vi "Struct Fill Cluster By Items Record.vi"(7 "reinit cluster to default (false)":bool, 8 "error in":errorcluster, 9 "data start offset (0)":i32, 10 "data in":u8[](array[numeric])=[9, 0, 0, 0, 15, 0, 0, 0, 1, 78, 0, 1, 0, 0, 0, 1, 0, 0, 0, 1, 0, 0, 0, 43, 0, 0, 0, 1, 97, 3, 1, 0, 0, 0, 4, 0, 0, 0, 0, 0, 0, 0, 0, 0, 240, 63, 0, 0, 0, 0, 0, 0, 0, 64, 0, 0, 0, 0, 0, 0, 8, 64, 0, 0, 0, 0, 0, 0, 16, 64, 43, 0, 0, 0, 1, 66, 3, 2, 0, 0, 0, 2, 0, 0, 0, 0, 0, 0, 0, 0, 0, 240, 63, 0, 0, 0, 0, 0, 0, 8, 64, 0, 0, 0, 0, 0, 0, 0, 64, 0, 0, 0, 0, 0, 0, 16, 64, 22, 0, 0, 0, 3, 115, 116, 114, 4, 1, 0, 0, 0, 9, 0, 0, 0, 100, 118, 101, 32, 104, 111, 118, 110, 111, 44, 0, 0, 0, 2, 99, 97, 131, 2, 0, 0, 0, 1, 0, 0, 0, 0, 0, 0, 0, 0, 0, 240, 63, 0, 0, 0, 0, 0, 0, 240, 63, 0, 0, 0, 0, 0, 0, 0, 64, 0, 0, 0, 0, 0, 0, 240, 191, 109, 0, 0, 0, 5, 115, 116, 114, 117, 99, 5, 1, 0, 0, 0, 1, 0, 0, 0, 3, 0, 0, 0, 16, 0, 0, 0, 3, 115, 116, 114, 4, 1, 0, 0, 0, 3, 0, 0, 0, 97, 115, 115, 19, 0, 0, 0, 1, 110, 3, 1, 0, 0, 0, 1, 0, 0, 0, 0, 0, 0, 0, 0, 128, 75, 64, 43, 0, 0, 0, 1, 65, 3, 2, 0, 0, 0, 2, 0, 0, 0, 0, 0, 0, 0, 0, 0, 240, 63, 0, 0, 0, 0, 0, 0, 8, 64, 0, 0, 0, 0, 0, 0, 0, 64, 0, 0, 0, 0, 0, 0, 16, 64, 218, 0, 0, 0, 2, 115, 118, 5, 1, 0, 0, 0, 2, 0, 0, 0, 3, 0, 0, 0, 16, 0, 0, 0, 3, 115, 116, 114, 4, 1, 0, 0, 0, 3, 0, 0, 0, 97, 115, 115, 19, 0, 0, 0, 1, 110, 3, 1, 0, 0, 0, 1, 0, 0, 0, 0, 0, 0, 0, 0, 128, 75, 64, 43, 0, 0, 0, 1, 65, 3, 2, 0, 0, 0, 2, 0, 0, 0, 0, 0, 0, 0, 0, 0, 240, 63, 0, 0, 0, 0, 0, 0, 8, 64, 0, 0, 0, 0, 0, 0, 0, 64, 0, 0, 0, 0, 0, 0, 16, 64, 3, 0, 0, 0, 34, 0, 0, 0, 3, 115, 116, 114, 4, 1, 0, 0, 0, 21, 0, 0, 0, 110, 101, 106, 97, 107, 101, 106, 32, 106, 105, 110, 101, 106, 32, 114, 101, 116, 101, 122, 101, 99, 19, 0, 0, 0, 1, 110, 3, 1, 0, 0, 0, 1, 0, 0, 0, 0, 0, 0, 0, 0, 0, 86, 64, 43, 0, 0, 0, 1, 65, 3, 2, 0, 0, 0, 2, 0, 0, 0, 0, 0, 0, 0, 0, 0, 240, 63, 0, 0, 0, 0, 0, 0, 8, 64, 0, 0, 0, 0, 0, 0, 0, 64, 0, 0, 0, 0, 0, 0, 16, 64, 132, 1, 0, 0, 2, 115, 99, 5, 2, 0, 0, 0, 2, 0, 0, 0, 3, 0, 0, 0, 16, 0, 0, 0, 3, 115, 116, 114, 4, 1, 0, 0, 0, 3, 0, 0, 0, 97, 115, 115, 19, 0, 0, 0, 1, 110, 3, 1, 0, 0, 0, 1, 0, 0, 0, 0, 0, 0, 0, 0, 128, 75, 64, 43, 0, 0, 0, 1, 65, 3, 2, 0, 0, 0, 2, 0, 0, 0, 0, 0, 0, 0, 0, 0, 240, 63, 0, 0, 0, 0, 0, 0, 8, 64, 0, 0, 0, 0, 0, 0, 0, 64, 0, 0, 0, 0, 0, 0, 16, 64, 3, 0, 0, 0, 16, 0, 0, 0, 3, 115, 116, 114, 4, 1, 0, 0, 0, 3, 0, 0, 0, 97, 115, 115, 19, 0, 0, 0, 1, 110, 3, 1, 0, 0, 0, 1, 0, 0, 0, 0, 0, 0, 0, 0, 128, 75, 64, 43, 0, 0, 0, 1, 65, 3, 2, 0, 0, 0, 2, 0, 0, 0, 0, 0, 0, 0, 0, 0, 240, 63, 0, 0, 0, 0, 0, 0, 8, 64, 0, 0, 0, 0, 0, 0, 0, 64, 0, 0, 0, 0, 0, 0, 16, 64, 3, 0, 0, 0, 16, 0, 0, 0, 3, 115, 116, 114, 4, 1, 0, 0, 0, 3, 0, 0, 0, 97, 115, 115, 19, 0, 0, 0, 1, 110, 3, 1, 0, 0, 0, 1, 0, 0, 0, 0, 0, 0, 0, 0, 128, 75, 64, 43, 0, 0, 0, 1, 65, 3, 2, 0, 0, 0, 2, 0, 0, 0, 0, 0, 0, 0, 0, 0, 240, 63, 0, 0, 0, 0, 0, 0, 8, 64, 0, 0, 0, 0, 0, 0, 0, 64, 0, 0, 0, 0, 0, 0, 16, 64, 3, 0, 0, 0, 16, 0, 0, 0, 3, 115, 116, 114, 4, 1, 0, 0, 0, 3, 0, 0, 0, 97, 115, 115, 19, 0, 0, 0, 1, 110, 3, 1, 0, 0, 0, 1, 0, 0, 0, 0, 0, 0, 0, 0, 128, 75, 64, 43, 0, 0, 0, 1, 65, 3, 2, 0, 0, 0, 2, 0, 0, 0, 0, 0, 0, 0, 0, 0, 240, 63, 0, 0, 0, 0, 0, 0, 8, 64, 0, 0, 0, 0, 0, 0, 0, 64, 0, 0, 0, 0, 0, 0, 16, 64, 26, 0, 0, 0, 4, 99, 115, 116, 114, 5, 1, 0, 0, 0, 3, 0, 0, 0, 0, 0, 0, 0, 0, 0, 0, 0, 0, 0, 0, 0], 11 "cluster ref (empty)":refnum<vi>) -> (0 "error out":errorcluster, 2 "octave struct out":T1[](array[typedef]), 3 "cluster ref out (copy)":refnum<vi>)   [LabVIEW 2013, in "GOLPI library.lvlib"]
doc: "This VI will use binary struct data generated by GNU Octave GOLPI function 'golpi_conv_struct()'. It will try to assign all elements from the Octave to the elements of matching names in the referenced cluser. Optionally it can reset the cluster default before. If it is called with invalid reference to the cluster it will just parse the binary data and return the items list. The function is recoursive so it should be able to assign clusters within clusters and so on."
uses:
  GOLPI library.lvlib
  Struct Item Record.ctl
  Struct Item Types.ctl
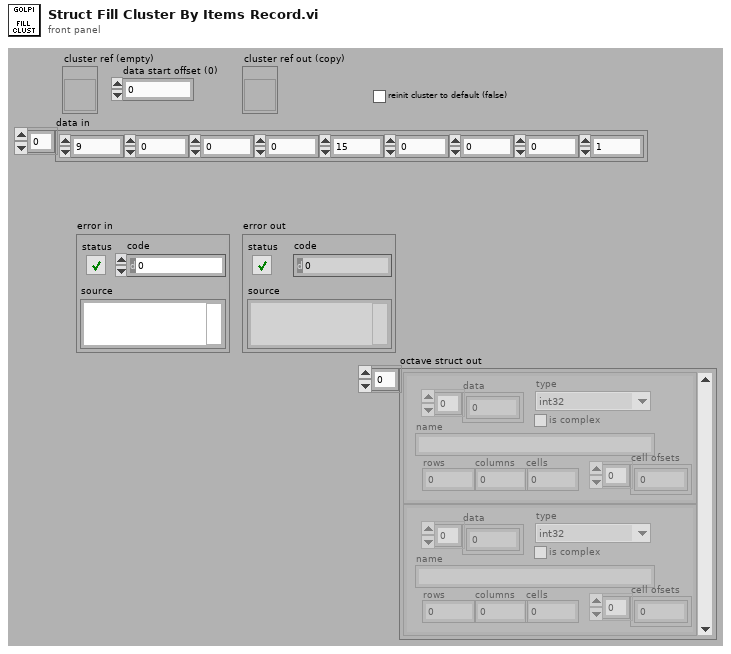
[diagram p1: front panel]
types:
  T1 = typedef "GOLPI library.lvlib/Struct Item Record.ctl" = cluster{"data":u8[], "type":T2, "name":string, "rows":i32, "columns":i32, "cells":i32, "is complex":bool, "cell ofsets":u32[]}
  T2 = typedef "GOLPI library.lvlib/Struct Item Types.ctl" = enum16{"int32", "uint32", "single", "double", "string", "cell array"}
  T3 = enum16{"big-endian, network order", "native, host order", "little-endian"}
  T4 = typedef "GOLPI library.lvlib/Struct Data Types.ctl" = enum16{"n/a", "Real", "Complex", "String/path", "Cluster", "Bool"}
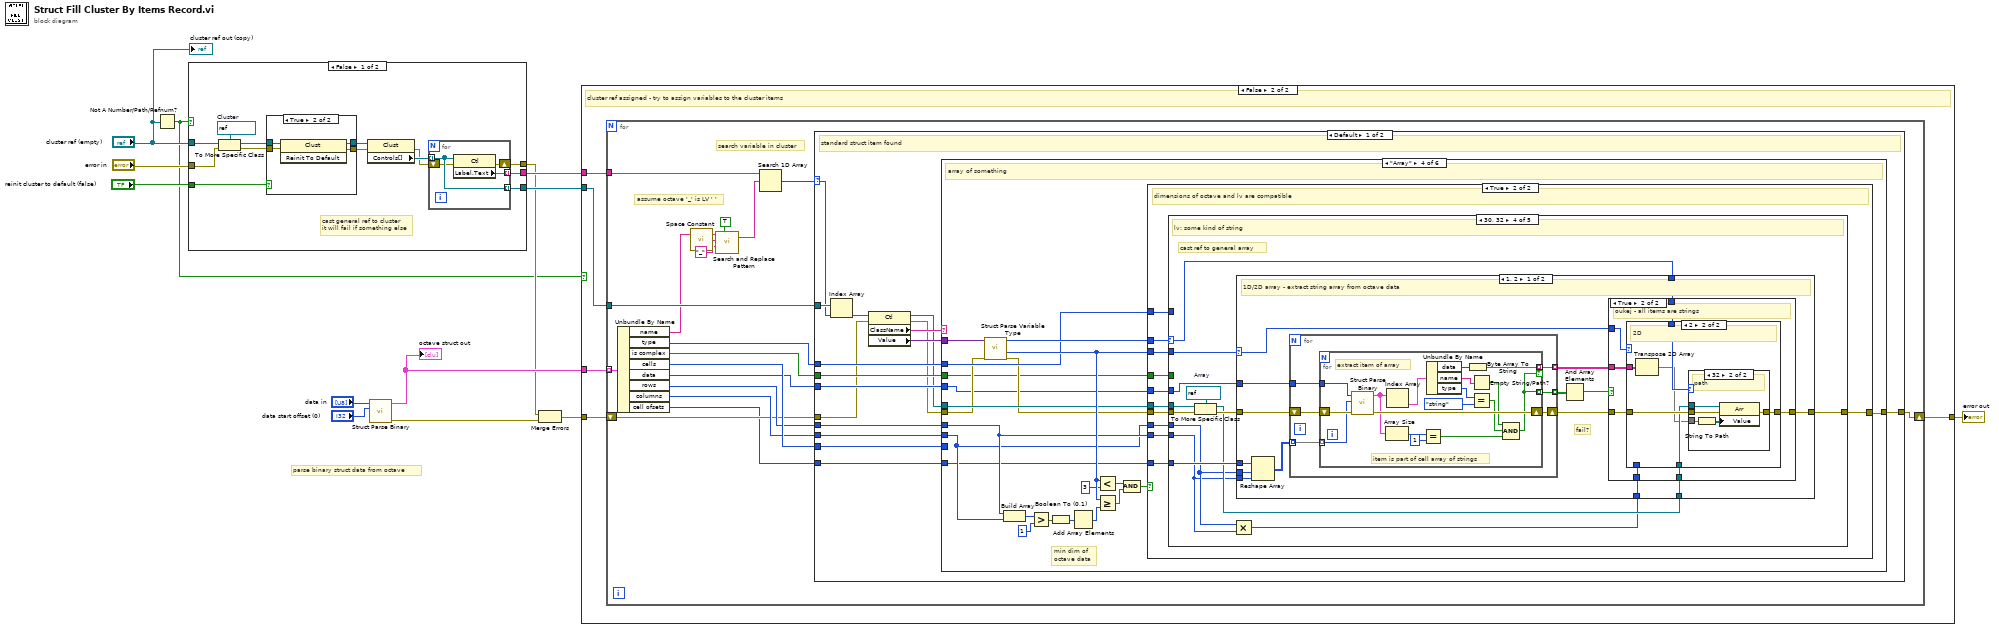
[diagram p0: block diagram]
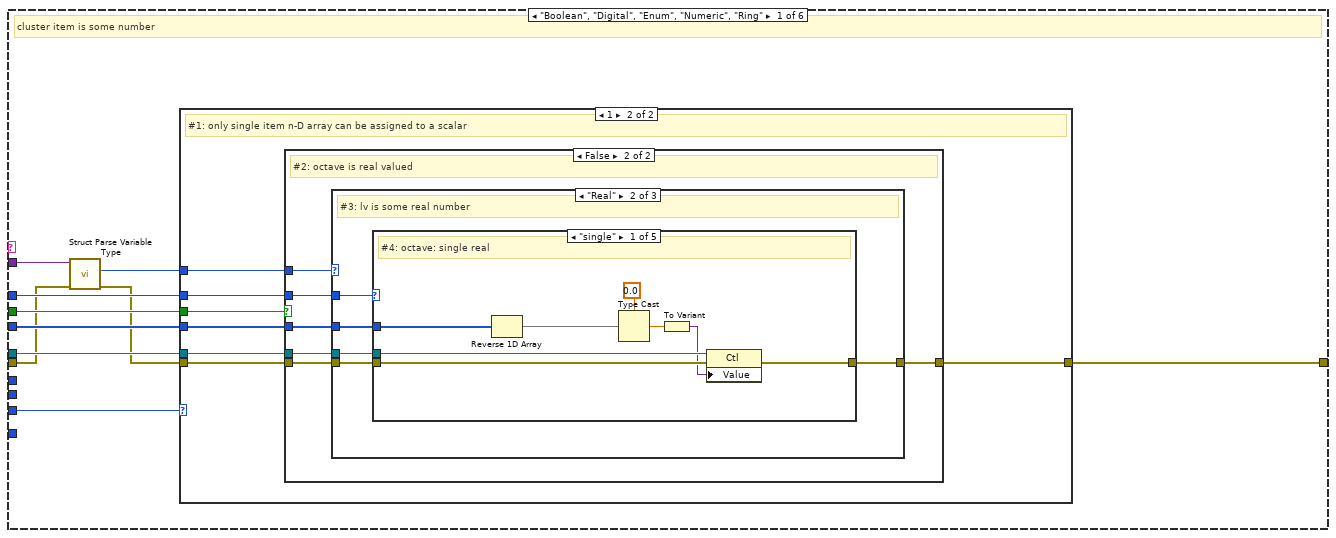
[diagram p3: hidden frame]
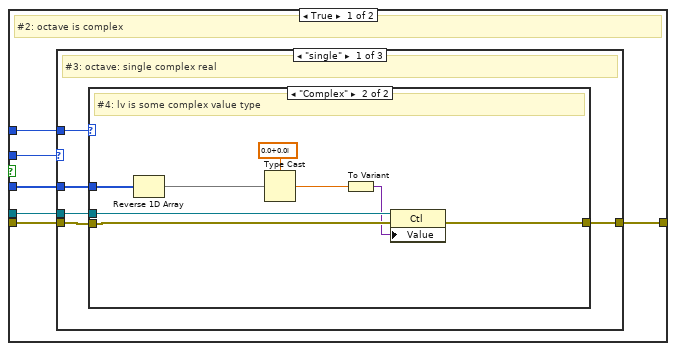
[diagram p5: hidden frame]
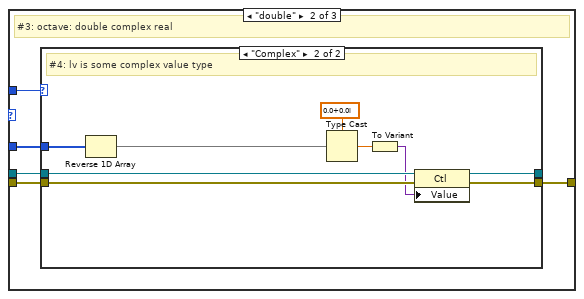
[diagram p7: hidden frame]
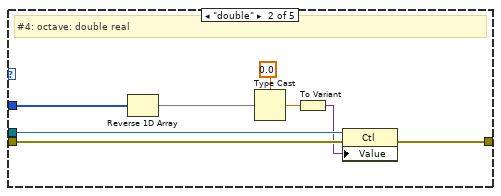
[diagram p11: hidden frame]
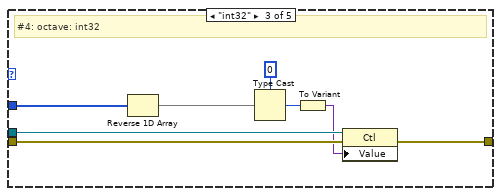
[diagram p12: hidden frame]
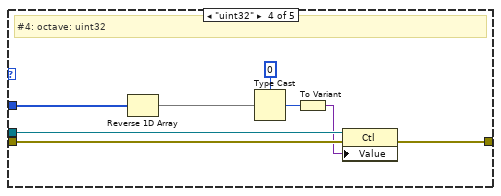
[diagram p13: hidden frame]
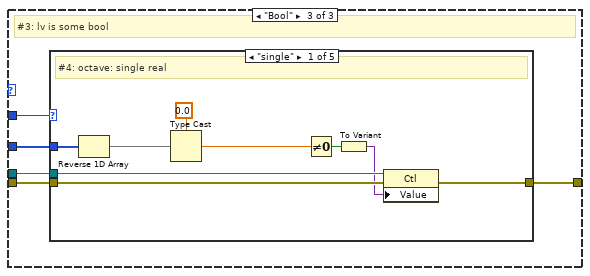
[diagram p15: hidden frame]
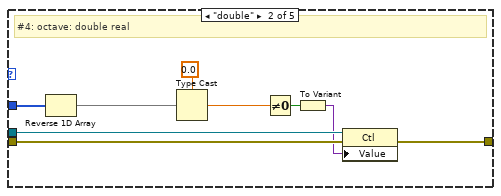
[diagram p16: hidden frame]
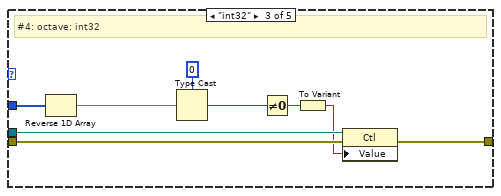
[diagram p17: hidden frame]
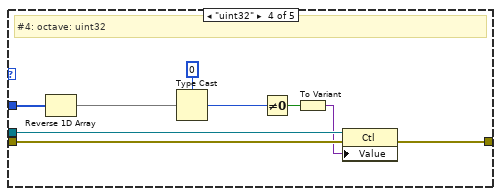
[diagram p18: hidden frame]
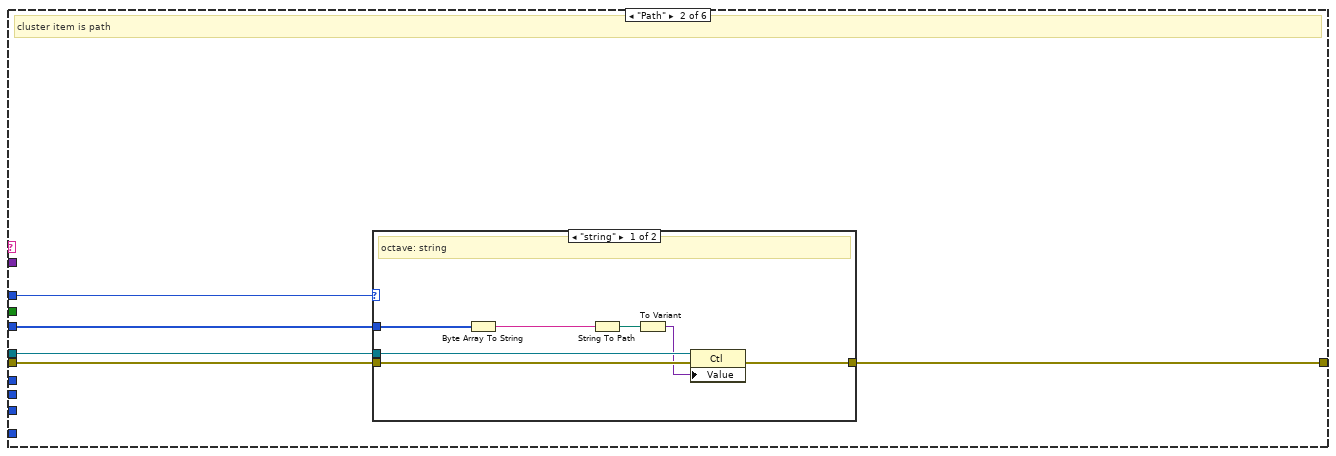
[diagram p20: hidden frame]
diagram:
  # "parse binary struct data from octave"
  n1 = Not A Number/Path/Refnum?(number/path/refnum="cluster ref (empty)") -> (NaN/Path/Refnum?=w1:bool)
  n2 = case shown="False" w1 {
    tunnel: [w25 _] -> w11
    tunnel: [w24 _] -> w10
    tunnel: "error in" -> [w22 w37]
    tunnel: "cluster ref (empty)" -> [w15 _]
    tunnel: "reinit cluster to default (false)" -> [w17 _]
    tunnel: [w14 w37] -> w4
    frame False {
      w23 = refnum<vi> refnum  # Cluster
      # "cast general ref to cluster\nit will fail if something else"
      n3 = To More Specific Class(target class=w23, reference=w15, error in=w22) -> (specific class reference=w19:refnum<vi>, error out=w18:errorcluster)
      n4 = case shown="True" w17 {
        tunnel: [w28 w32] -> w21
        tunnel: [w27 w31] -> w20
        tunnel: w19 -> [w27 w30]
        tunnel: w18 -> [w28 w29]
        frame False {
        }
        frame True {
          n5 = invoke class="Clust" method="Reinit To Default"(reference=w30, error in=w29) -> (reference out=w31:refnum<vi>, error out=w32:errorcluster)  [unwired: 1 in, 1 out]
        }
      }
      n6 = property class="Clust"(reference=w20, error in=w21) -> (error out=w16:errorcluster, "Controls[]"=w26:refnum<vi>[])  [unwired: 1 out]
      n7 = for {
        tunnel: w26 -> [w35] mode=indexing
        tunnel: [w36] -> w25 mode=indexing
        tunnel: [w35] -> w24 mode=indexing
        shift-right: [w33] -> w14
        shift-left: w16 -> [w34]
        n8 = property class="Ctl"(reference=w35, error in=w34) -> (error out=w33:errorcluster, "Label.Text"=w36:string)  [unwired: 1 out]
      }
    }
    frame True {
    }
  }
  n9 = call "Struct Parse Binary.vi"("data start offset (0)"="data start offset (0)", "data in"="data in") -> ("error out"=w3:errorcluster, "struct items"=w12:T1[])  [unwired: 8 in]
  "octave struct out" <- w12
  n10 = Merge Errors(w4, w3) -> (w2:errorcluster)
  n11 = case shown="False" w1 {
    tunnel: w12 -> [_ w43]
    tunnel: w11 -> [_ w42]
    tunnel: w10 -> [_ w41]
    tunnel: [w38 w40] -> w9
    tunnel: w2 -> [w38 w39]
    frame True {
      # "no cluster ref assigned - skip assigning, just parse struct"
    }
    frame False {
      # "cluster ref assigned - try to assign variables to the cluster items"
      n12 = for {
        tunnel: w43 -> [w61] mode=indexing
        tunnel: w42 -> [w60]
        tunnel: w41 -> [w59]
        shift-right: [w52] -> w40
        shift-left: w39 -> [w51]
        # "assume octave '_' is LV ' '"
        # "search variable in cluster"
        n13 = Unbundle By Name(w61) -> ("name"=w48:string, "type"=w58:T2, "is complex"=w57:bool, "cells"=w56:i32, "data"=w55:u8[], "rows"=w54:i32, "columns"=w53:i32, "cell ofsets"=w50:u32[])
        n14 = call <vilib>:"Space Constant.vi"() -> ("String"=w44:string)
        n15 = call <vilib>:"Search and Replace Pattern.vi"("string"=w48, "regular expression (\"\")"="_", "replace string (\"\")"=w44, "replace all? (F)"=TRUE) -> ("result string"=w47:string)  [unwired: 1 in, 1 out]
        n16 = Search 1D Array(1D array=w60, element=w47) -> (index of element=w49:i32)  [unwired: 1 in]
        n17 = case shown="Default" w49 {
          selector: w49 -> [w76 _]
          tunnel: w59 -> [w77 _]
          tunnel: w58 -> [w72 _]
          tunnel: w57 -> [w71 _]
          tunnel: w56 -> [w70 _]
          tunnel: w55 -> [w69 _]
          tunnel: w54 -> [w66 _]
          tunnel: w53 -> [w65 _]
          tunnel: [w64 w626] -> w52
          tunnel: w51 -> [w63 w626]
          tunnel: w50 -> [w62 _]
          frame Default {
            # "standard struct item found"
            n18 = Index Array(array=w77, index=w76) -> (element=w75:refnum<vi>)
            n19 = property class="Ctl"(reference=w75, error in=w63) -> (reference out=w68:refnum<vi>, error out=w67:errorcluster, "ClassName"=w74:string, "Value"=w73:variant)
            n20 = case shown="\"Array\"" w74 {
              tunnel: w73 -> [w87 _ _ w246 _ _]
              tunnel: w72 -> [w86 w224 w237 w253 w613 _]
              tunnel: w71 -> [w82 _ _ w250 _ _]
              tunnel: w70 -> [w83 _ _ _ w615 _]
              tunnel: w69 -> [w85 w223 w236 w249 w607 _]
              tunnel: w68 -> [w81 w222 w235 w255 w608 _]
              tunnel: w67 -> [w79 w221 w234 w252 w616 w625]
              tunnel: [w80 w220 w233 w256 w606 w625] -> w64
              tunnel: w66 -> [_ _ _ w248 _ _]
              tunnel: w65 -> [_ _ _ w247 _ _]
              tunnel: w62 -> [_ _ _ w245 _ _]
              frame "Boolean", "Digital", "Enum", "Numeric", "Ring" {
                # "cluster item is some number"
                n21 = call "Struct Parse Variable Type.vi"("error in"=w79, "variant in"=w87) -> ("error out"=w78:errorcluster, "data type"=w84:T4)  [unwired: 6 in, 2 out]
                n22 = case shown="1" w83 {
                  tunnel: w86 -> [_ w95]
                  tunnel: w85 -> [_ w94]
                  tunnel: w84 -> [_ w93]
                  tunnel: w82 -> [_ w92]
                  tunnel: w81 -> [_ w91]
                  tunnel: w78 -> [w88 w90]
                  tunnel: [w88 w89] -> w80
                  frame Default {
                    # "error - can't assign multi cell array to a scalar"
                  }
                  frame 1 {
                    # "#1: only single item n-D array can be assigned to a scalar"
                    n23 = case shown="False" w92 {
                      tunnel: w95 -> [w101 w138]
                      tunnel: w94 -> [w100 w137]
                      tunnel: w93 -> [w99 w133]
                      tunnel: w91 -> [w98 w136]
                      tunnel: w90 -> [w97 w135]
                      tunnel: [w96 w134] -> w89
                      frame True {
                        # "#2: octave is complex"
                        n24 = case shown="\"single\"" w101 {
                          tunnel: w100 -> [w105 w119 _]
                          tunnel: w99 -> [w106 w120 _]
                          tunnel: w98 -> [w104 w118 _]
                          tunnel: w97 -> [w103 w117 w132]
                          tunnel: [w102 w116 w132] -> w96
                          frame "single" {
                            # "#3: octave: single complex real"
                            n25 = case shown="\"Complex\"" w106 {
                              tunnel: w105 -> [_ w115]
                              tunnel: w104 -> [_ w112]
                              tunnel: w103 -> [w107 w111]
                              tunnel: [w107 w108] -> w102
                              frame Default {
                                # "#4: error: invalid octave type"
                              }
                              frame "Complex" {
                                # "#4: lv is some complex value type"
                                n26 = Reverse 1D Array(array=w115) -> (reversed array=w114:u8[])
                                n27 = Type Cast(type=csg 0.0+0.0i, x=w114) -> (*(type *) &x=w110:csg)
                                n28 = To Variant(anything=w110) -> (Variant=w109:variant)
                                n29 = property class="Ctl"(reference=w112, error in=w111, "Value"=w109) -> (error out=w108:errorcluster)  [unwired: 1 out]
                              }
                            }
                          }
                          frame "double" {
                            # "#3: octave: double complex real"
                            n30 = case shown="\"Complex\"" w120 {
                              tunnel: w119 -> [_ w131]
                              tunnel: w118 -> [w121 w128]
                              tunnel: w117 -> [w122 w127]
                              tunnel: [w122 w124] -> w116
                              tunnel: [w121 w123] -> _
                              frame Default {
                              }
                              frame "Complex" {
                                # "#4: lv is some complex value type"
                                n31 = Reverse 1D Array(array=w131) -> (reversed array=w130:u8[])
                                n32 = Type Cast(type=cdb 0.0+0.0i, x=w130) -> (*(type *) &x=w126:cdb)
                                n33 = To Variant(anything=w126) -> (Variant=w125:variant)
                                n34 = property class="Ctl"(reference=w128, error in=w127, "Value"=w125) -> (reference out=w123:refnum<vi>, error out=w124:errorcluster)
                              }
                            }
                          }
                          frame Default {
                            # "#3: invalid octave type"
                          }
                        }
                      }
                      frame False {
                        # "#2: octave is real valued"
                        n35 = case shown="\"Real\"" w133 {
                          tunnel: w138 -> [_ w144 w182]
                          tunnel: w137 -> [_ w143 w181]
                          tunnel: w136 -> [_ w142 w180]
                          tunnel: w135 -> [w139 w141 w179]
                          tunnel: [w139 w140 w178] -> w134
                          frame Default {
                            # "#3: bad lv type"
                          }
                          frame "Real" {
                            # "#3: lv is some real number"
                            n36 = case shown="\"single\"" w144 {
                              tunnel: w143 -> [w152 w160 w168 w176 _]
                              tunnel: w142 -> [w151 w159 w167 w175 _]
                              tunnel: w141 -> [w150 w158 w166 w174 w177]
                              tunnel: [w149 w157 w165 w173 w177] -> w140
                              frame "single" {
                                # "#4: octave: single real"
                                n37 = Reverse 1D Array(array=w152) -> (reversed array=w148:u8[])
                                n38 = Type Cast(type=sgl 0.0, x=w148) -> (*(type *) &x=w146:sgl)
                                n39 = To Variant(anything=w146) -> (Variant=w145:variant)
                                n40 = property class="Ctl"(reference=w151, error in=w150, "Value"=w145) -> (error out=w149:errorcluster)  [unwired: 1 out]
                              }
                              frame "double" {
                                # "#4: octave: double real"
                                n41 = Reverse 1D Array(array=w160) -> (reversed array=w156:u8[])
                                n42 = Type Cast(type=0.0, x=w156) -> (*(type *) &x=w154:dbl)
                                n43 = To Variant(anything=w154) -> (Variant=w153:variant)
                                n44 = property class="Ctl"(reference=w159, error in=w158, "Value"=w153) -> (error out=w157:errorcluster)  [unwired: 1 out]
                              }
                              frame "int32" {
                                # "#4: octave: int32"
                                n45 = Reverse 1D Array(array=w168) -> (reversed array=w164:u8[])
                                n46 = Type Cast(type=0, x=w164) -> (*(type *) &x=w162:i32)
                                n47 = To Variant(anything=w162) -> (Variant=w161:variant)
                                n48 = property class="Ctl"(reference=w167, error in=w166, "Value"=w161) -> (error out=w165:errorcluster)  [unwired: 1 out]
                              }
                              frame "uint32" {
                                # "#4: octave: uint32"
                                n49 = Reverse 1D Array(array=w176) -> (reversed array=w172:u8[])
                                n50 = Type Cast(type=u32 0, x=w172) -> (*(type *) &x=w170:u32)
                                n51 = To Variant(anything=w170) -> (Variant=w169:variant)
                                n52 = property class="Ctl"(reference=w175, error in=w174, "Value"=w169) -> (error out=w173:errorcluster)  [unwired: 1 out]
                              }
                              frame Default {
                                # "#4: invalid octave type"
                              }
                            }
                          }
                          frame "Bool" {
                            # "#3: lv is some bool"
                            n53 = case shown="\"single\"" w182 {
                              tunnel: w181 -> [w191 w200 w209 w218 _]
                              tunnel: w180 -> [w190 w199 w208 w217 _]
                              tunnel: w179 -> [w189 w198 w207 w216 w219]
                              tunnel: [w188 w197 w206 w215 w219] -> w178
                              frame "single" {
                                # "#4: octave: single real"
                                n54 = Reverse 1D Array(array=w191) -> (reversed array=w187:u8[])
                                n55 = Type Cast(type=sgl 0.0, x=w187) -> (*(type *) &x=w185:sgl)
                                n56 = Not Equal To 0?(x=w185) -> (x != 0?=w183:bool)
                                n57 = To Variant(anything=w183) -> (Variant=w184:variant)
                                n58 = property class="Ctl"(reference=w190, error in=w189, "Value"=w184) -> (error out=w188:errorcluster)  [unwired: 1 out]
                              }
                              frame "double" {
                                # "#4: octave: double real"
                                n59 = Reverse 1D Array(array=w200) -> (reversed array=w196:u8[])
                                n60 = Type Cast(type=0.0, x=w196) -> (*(type *) &x=w194:dbl)
                                n61 = Not Equal To 0?(x=w194) -> (x != 0?=w192:bool)
                                n62 = To Variant(anything=w192) -> (Variant=w193:variant)
                                n63 = property class="Ctl"(reference=w199, error in=w198, "Value"=w193) -> (error out=w197:errorcluster)  [unwired: 1 out]
                              }
                              frame "int32" {
                                # "#4: octave: int32"
                                n64 = Reverse 1D Array(array=w209) -> (reversed array=w205:u8[])
                                n65 = Type Cast(type=0, x=w205) -> (*(type *) &x=w203:i32)
                                n66 = Not Equal To 0?(x=w203) -> (x != 0?=w201:bool)
                                n67 = To Variant(anything=w201) -> (Variant=w202:variant)
                                n68 = property class="Ctl"(reference=w208, error in=w207, "Value"=w202) -> (error out=w206:errorcluster)  [unwired: 1 out]
                              }
                              frame "uint32" {
                                # "#4: octave: uint32"
                                n69 = Reverse 1D Array(array=w218) -> (reversed array=w214:u8[])
                                n70 = Type Cast(type=u32 0, x=w214) -> (*(type *) &x=w212:u32)
                                n71 = Not Equal To 0?(x=w212) -> (x != 0?=w210:bool)
                                n72 = To Variant(anything=w210) -> (Variant=w211:variant)
                                n73 = property class="Ctl"(reference=w217, error in=w216, "Value"=w211) -> (error out=w215:errorcluster)  [unwired: 1 out]
                              }
                              frame Default {
                                # "#4: invalid octave type"
                              }
                            }
                          }
                        }
                      }
                    }
                  }
                }
              }
              frame "Path" {
                # "cluster item is path"
                n74 = case shown="\"string\"" w224 {
                  tunnel: w223 -> [w227 _]
                  tunnel: w222 -> [w231 _]
                  tunnel: w221 -> [w230 w232]
                  tunnel: [w229 w232] -> w220
                  frame "string" {
                    # "octave: string"
                    n75 = Byte Array To String(unsigned byte array=w227) -> (string=w226:string)
                    n76 = String To Path(string=w226) -> (path=w225:path)
                    n77 = To Variant(anything=w225) -> (Variant=w228:variant)
                    n78 = property class="Ctl"(reference=w231, error in=w230, "Value"=w228) -> (error out=w229:errorcluster)  [unwired: 1 out]
                  }
                  frame Default {
                    # "error: invalid octave type"
                  }
                }
              }
              frame "ComboBox", "DAQmxName", "IVILogicalName", "IVIResourceName", "String", "VISAResourceName" {
                # "cluster item is some string type"
                n79 = case shown="\"string\"" w237 {
                  tunnel: w236 -> [w239 _]
                  tunnel: w235 -> [w243 _]
                  tunnel: w234 -> [w242 w244]
                  tunnel: [w241 w244] -> w233
                  frame "string" {
                    # "octave: string"
                    n80 = Byte Array To String(unsigned byte array=w239) -> (string=w238:string)
                    n81 = To Variant(anything=w238) -> (Variant=w240:variant)
                    n82 = property class="Ctl"(reference=w243, error in=w242, "Value"=w240) -> (error out=w241:errorcluster)  [unwired: 1 out]
                  }
                  frame Default {
                    # "error: invalid octave type"
                  }
                }
              }
              frame "Array" {
                # "min dim of\noctave data"
                # "array of something"
                n83 = call "Struct Parse Variable Type.vi"("error in"=w252, "variant in"=w246) -> ("error out"=w251:errorcluster, "array dims"=w261:i16, "type id"=w254:i16)  [unwired: 6 in, 1 out]
                n84 = Build Array(w248, w247) -> (w266:i32[])
                n85 = Greater?(x=w266, y=1) -> (0:w264:bool[])
                n86 = Boolean To (0,1)(Boolean=w264) -> (0, 1=w263:i16[])
                n87 = Add Array Elements(numeric array=w263) -> (sum=w262:i16)
                n88 = Less?(x=w261, y=i16 3) -> (x < y?=w259:bool)
                n89 = Greater Or Equal?(x=w261, y=w262) -> (x >= y?=w258:bool)
                n90 = Compound Arithmetic op=AND(w259, w258) -> (w257:bool)
                n91 = case shown="True" w257 {
                  tunnel: w254 -> [_ w278]
                  tunnel: w261 -> [_ w277]
                  tunnel: [w267 w271] -> w256
                  tunnel: w251 -> [w267 w275]
                  tunnel: w255 -> [_ w274]
                  tunnel: w253 -> [_ w276]
                  tunnel: w250 -> [_ w273]
                  tunnel: w249 -> [_ w272]
                  tunnel: w247 -> [_ w270]
                  tunnel: w248 -> [_ w269]
                  tunnel: w245 -> [_ w268]
                  frame False {
                    # "incompatible lv and octave dims"
                  }
                  frame True {
                    # "dimensions of octave and lv are compatible"
                    n92 = case shown="30, 32" w278 {
                      selector: w278 -> [_ _ _ w515 _]
                      tunnel: w277 -> [w281 w388 w453 w521 _]
                      tunnel: w276 -> [w287 w394 _ _ _]
                      tunnel: w275 -> [w286 w393 w466 w525 w605]
                      tunnel: w274 -> [w285 w392 w467 w526 _]
                      tunnel: w273 -> [w284 w391 _ _ _]
                      tunnel: w272 -> [w283 w390 w464 w523 _]
                      tunnel: [w282 w389 w454 w514 w605] -> w271
                      tunnel: w270 -> [w280 w387 w461 w518 _]
                      tunnel: w269 -> [w279 w386 w462 w517 _]
                      tunnel: w268 -> [_ _ w463 w522 _]
                      frame 1..11, 21..23 {
                        # "lv: real numerics"
                        n93 = case shown="False" w284 {
                          tunnel: w287 -> [w295 _]
                          tunnel: w286 -> [w294 w385]
                          tunnel: w285 -> [w291 _]
                          tunnel: w283 -> [w293 _]
                          tunnel: [w292 w385] -> w282
                          tunnel: w281 -> [w290 _]
                          tunnel: w280 -> [w289 _]
                          tunnel: w279 -> [w288 _]
                          frame False {
                            # "octave: real"
                            n94 = case shown="\"uint32\"" w295 {
                              tunnel: w294 -> [w298 w320 w342 w364 w384]
                              tunnel: w293 -> [w297 w319 w341 w363 _]
                              tunnel: [w305 w327 w349 w371 w384] -> w292
                              tunnel: w291 -> [w306 w328 w350 w372 _]
                              tunnel: w290 -> [w303 w325 w347 w369 _]
                              tunnel: w289 -> [w301 w323 w345 w367 _]
                              tunnel: w288 -> [w300 w322 w344 w366 _]
                              frame "int32" {
                                # "octave: int32 array"
                                n95 = Byte Array To String(unsigned byte array=w297) -> (string=w296:string)
                                n96 = Unflatten From String(type=i32[] [], binary string=w296, data includes array or string size? (T)=FALSE ("prepend array or string size? (T)"), byte order (0:big-endian, network order)=T3."little-endian", error in (no error)=w298) -> (value=w304:i32[], error out=w307:errorcluster)  [unwired: 1 out]
                                n97 = case shown="2" w303 {
                                tunnel: w304 -> [w310 w317]
                                tunnel: [w311 w315] -> w302
                                tunnel: w301 -> [_ w314]
                                tunnel: w300 -> [_ w313]
                                frame Default {
                                # "1D"
                                n98 = To Variant(anything=w310) -> (Variant=w311:variant)
                                }
                                frame 2 {
                                # "2D"
                                n99 = Reshape Array(w317, w314, w313) -> (w316:i32[][])
                                n100 = Transpose 2D Array(2D array=w316) -> (transposed array=w312:i32[][])
                                n101 = To Variant(anything=w312) -> (Variant=w315:variant)
                                }
                                }
                                n102 = property class="Ctl"(reference=w306, error in=w307, "Value"=w302) -> (error out=w305:errorcluster)  [unwired: 1 out]
                              }
                              frame "uint32" {
                                # "octave: uint32 array"
                                n103 = Byte Array To String(unsigned byte array=w319) -> (string=w318:string)
                                n104 = Unflatten From String(type=u32[] [], binary string=w318, data includes array or string size? (T)=FALSE ("prepend array or string size? (T)"), byte order (0:big-endian, network order)=T3."little-endian", error in (no error)=w320) -> (value=w326:u32[], error out=w329:errorcluster)  [unwired: 1 out]
                                n105 = case shown="2" w325 {
                                tunnel: w326 -> [w332 w339]
                                tunnel: [w333 w337] -> w324
                                tunnel: w323 -> [_ w336]
                                tunnel: w322 -> [_ w335]
                                frame Default {
                                # "1D"
                                n106 = To Variant(anything=w332) -> (Variant=w333:variant)
                                }
                                frame 2 {
                                # "2D"
                                n107 = Reshape Array(w339, w336, w335) -> (w338:u32[][])
                                n108 = Transpose 2D Array(2D array=w338) -> (transposed array=w334:u32[][])
                                n109 = To Variant(anything=w334) -> (Variant=w337:variant)
                                }
                                }
                                n110 = property class="Ctl"(reference=w328, error in=w329, "Value"=w324) -> (error out=w327:errorcluster)  [unwired: 1 out]
                              }
                              frame "single" {
                                # "octave: single real array"
                                n111 = Byte Array To String(unsigned byte array=w341) -> (string=w340:string)
                                n112 = Unflatten From String(type=sgl[] [], binary string=w340, data includes array or string size? (T)=FALSE ("prepend array or string size? (T)"), byte order (0:big-endian, network order)=T3."little-endian", error in (no error)=w342) -> (value=w348:sgl[], error out=w351:errorcluster)  [unwired: 1 out]
                                n113 = case shown="2" w347 {
                                tunnel: w348 -> [w354 w361]
                                tunnel: [w355 w359] -> w346
                                tunnel: w345 -> [_ w358]
                                tunnel: w344 -> [_ w357]
                                frame Default {
                                # "1D"
                                n114 = To Variant(anything=w354) -> (Variant=w355:variant)
                                }
                                frame 2 {
                                # "2D"
                                n115 = Reshape Array(w361, w358, w357) -> (w360:sgl[][])
                                n116 = Transpose 2D Array(2D array=w360) -> (transposed array=w356:sgl[][])
                                n117 = To Variant(anything=w356) -> (Variant=w359:variant)
                                }
                                }
                                n118 = property class="Ctl"(reference=w350, error in=w351, "Value"=w346) -> (error out=w349:errorcluster)  [unwired: 1 out]
                              }
                              frame "double" {
                                # "octave: double real array"
                                n119 = Byte Array To String(unsigned byte array=w363) -> (string=w362:string)
                                n120 = Unflatten From String(type=dbl[] [], binary string=w362, data includes array or string size? (T)=FALSE ("prepend array or string size? (T)"), byte order (0:big-endian, network order)=T3."little-endian", error in (no error)=w364) -> (value=w370:dbl[], error out=w373:errorcluster)  [unwired: 1 out]
                                n121 = case shown="2" w369 {
                                tunnel: w370 -> [w376 w383]
                                tunnel: [w377 w381] -> w368
                                tunnel: w367 -> [_ w380]
                                tunnel: w366 -> [_ w379]
                                frame Default {
                                # "1D"
                                n122 = To Variant(anything=w376) -> (Variant=w377:variant)
                                }
                                frame 2 {
                                # "2D"
                                n123 = Reshape Array(w383, w380, w379) -> (w382:dbl[][])
                                n124 = Transpose 2D Array(2D array=w382) -> (transposed array=w378:dbl[][])
                                n125 = To Variant(anything=w378) -> (Variant=w381:variant)
                                }
                                }
                                n126 = property class="Ctl"(reference=w372, error in=w373, "Value"=w368) -> (error out=w371:errorcluster)  [unwired: 1 out]
                              }
                              frame Default {
                                # "error: unknown"
                              }
                            }
                          }
                          frame True {
                            # "not allowed complexes"
                          }
                        }
                      }
                      frame 12..14 {
                        # "lv: complex numerics"
                        n127 = case shown="True" w391 {
                          tunnel: w394 -> [w402 _]
                          tunnel: w393 -> [w401 w448]
                          tunnel: w392 -> [w398 _]
                          tunnel: w390 -> [w400 _]
                          tunnel: [w399 w448] -> w389
                          tunnel: w388 -> [w397 _]
                          tunnel: w387 -> [w396 _]
                          tunnel: w386 -> [w395 _]
                          frame True {
                            # "octave: complex"
                            n128 = case shown="\"single\"" w402 {
                              tunnel: w401 -> [w405 w427 w447]
                              tunnel: w400 -> [w404 w426 _]
                              tunnel: [w412 w434 w447] -> w399
                              tunnel: w398 -> [w413 w435 _]
                              tunnel: w397 -> [w410 w432 _]
                              tunnel: w396 -> [w408 w430 _]
                              tunnel: w395 -> [w407 w429 _]
                              frame "single" {
                                # "octave: single real array"
                                n129 = Byte Array To String(unsigned byte array=w404) -> (string=w403:string)
                                n130 = Unflatten From String(type=csg[] [], binary string=w403, data includes array or string size? (T)=FALSE ("prepend array or string size? (T)"), byte order (0:big-endian, network order)=T3."little-endian", error in (no error)=w405) -> (value=w411:csg[], error out=w414:errorcluster)  [unwired: 1 out]
                                n131 = case shown="2" w410 {
                                tunnel: w411 -> [w417 w424]
                                tunnel: [w418 w423] -> w409
                                tunnel: w408 -> [_ w422]
                                tunnel: w407 -> [_ w421]
                                frame Default {
                                # "1D"
                                n132 = To Variant(anything=w417) -> (Variant=w418:variant)
                                }
                                frame 2 {
                                # "2D"
                                n133 = Reshape Array(w424, w422, w421) -> (w420:csg[][])
                                n134 = Transpose 2D Array(2D array=w420) -> (transposed array=w419:csg[][])
                                n135 = To Variant(anything=w419) -> (Variant=w423:variant)
                                }
                                }
                                n136 = property class="Ctl"(reference=w413, error in=w414, "Value"=w409) -> (error out=w412:errorcluster)  [unwired: 1 out]
                              }
                              frame "double" {
                                # "octave: double real array"
                                n137 = Byte Array To String(unsigned byte array=w426) -> (string=w425:string)
                                n138 = Unflatten From String(type=cdb[] [], binary string=w425, data includes array or string size? (T)=FALSE ("prepend array or string size? (T)"), byte order (0:big-endian, network order)=T3."little-endian", error in (no error)=w427) -> (value=w433:cdb[], error out=w436:errorcluster)  [unwired: 1 out]
                                n139 = case shown="2" w432 {
                                tunnel: w433 -> [w439 w446]
                                tunnel: [w440 w445] -> w431
                                tunnel: w430 -> [_ w444]
                                tunnel: w429 -> [_ w443]
                                frame Default {
                                # "1D"
                                n140 = To Variant(anything=w439) -> (Variant=w440:variant)
                                }
                                frame 2 {
                                # "2D"
                                n141 = Reshape Array(w446, w444, w443) -> (w442:cdb[][])
                                n142 = Transpose 2D Array(2D array=w442) -> (transposed array=w441:cdb[][])
                                n143 = To Variant(anything=w441) -> (Variant=w445:variant)
                                }
                                }
                                n144 = property class="Ctl"(reference=w435, error in=w436, "Value"=w431) -> (error out=w434:errorcluster)  [unwired: 1 out]
                              }
                              frame Default {
                                # "error: invalid octave data"
                              }
                            }
                          }
                          frame False {
                            # "not allowed reals"
                          }
                        }
                      }
                      frame 80 {
                        w449 = u32 1 ("Number of Columns")
                        w465 = refnum<vi> refnum  # Array
                        # "restore original visible size"
                        # "set visible array size to [1,1]\n###todo: probably unnecessary\nbut without this indexing never works\nas it shoudl, it sometimes writes to [+1;+1] offset"
                        # "cast ref to general array"
                        # "clear array first\n###todo: this is fucked up way\nbecause it may have some \ndata as default but I found\nno better way"
                        # "lv: cluster"
                        n145 = To More Specific Class(target class=w465, reference=w467, error in=w466) -> (specific class reference=w459:refnum<vi>, error out=w460:errorcluster)
                        n146 = invoke class="Arr" method="Reinit To Default"(reference=w459, error in=w460) -> (reference out=w457:refnum<vi>, error out=w458:errorcluster)  [unwired: 1 in, 1 out]
                        n147 = property class="Arr"(reference=w457, error in=w458, "Number of Columns"=w449, "Number of Rows"=w449) -> (reference out=w450:refnum<vi>, error out=w456:errorcluster, "Number of Columns"=w452:u32, "Number of Rows"=w451:u32)
                        n148 = case shown="2" w453 {
                          tunnel: [w472 w492 w513] -> w455
                          tunnel: w464 -> [w471 w491 _]
                          tunnel: w463 -> [w468 w490 _]
                          tunnel: w462 -> [_ w489 _]
                          tunnel: w461 -> [_ w488 _]
                          tunnel: w456 -> [w470 w486 w513]
                          tunnel: w450 -> [w469 w485 _]
                          frame 1 {
                            # "1D array"
                            n149 = for {
                              tunnel: w469 -> [w480]
                              shift-right: [w477] -> w472
                              shift-left: w470 -> [w481]
                              tunnel: w471 -> [w475]
                              tunnel: w468 -> [w474] mode=indexing
                              i -> [w473]
                              w483 = refnum<vi> refnum  # Cluster
                              n150 = Build Array(w473) -> (w479:i32[])
                              n151 = property class="Arr"(reference=w480, error in=w481, "Index Values"=w479) -> (error out=w484:errorcluster, "Array Element"=w482:refnum<vi>)  [unwired: 1 out]
                              n152 = To More Specific Class(target class=w483, reference=w482, error in=w484) -> (specific class reference=w476:refnum<vi>, error out=w478:errorcluster)
                              n153 = call "Struct Fill Cluster By Items Record.vi"("error in"=w478, "data start offset (0)"=w474, "data in"=w475, "cluster ref (empty)"=w476) -> ("error out"=w477:errorcluster)  [unwired: 5 in, 2 out]
                            }
                          }
                          frame 2 {
                            # "2D array"
                            n154 = Reshape Array(w490, w488, w489) -> (w487:u32[][])
                            n155 = for {
                              tunnel: w485 -> [w498]
                              shift-right: [w497] -> w492
                              shift-left: w486 -> [w496]
                              tunnel: w491 -> [w494]
                              tunnel: w487 -> [w493] mode=indexing
                              i -> [w495]
                              n156 = for {
                                tunnel: w498 -> [w508]
                                shift-right: [w505] -> w497
                                shift-left: w496 -> [w509]
                                tunnel: w495 -> [w500]
                                tunnel: w494 -> [w503]
                                tunnel: w493 -> [w502] mode=indexing
                                i -> [w501]
                                w511 = refnum<vi> refnum  # Cluster
                                n157 = Build Array(w501, w500) -> (w507:i32[])
                                n158 = property class="Arr"(reference=w508, error in=w509, "Index Values"=w507) -> (error out=w512:errorcluster, "Array Element"=w510:refnum<vi>)  [unwired: 1 out]
                                n159 = To More Specific Class(target class=w511, reference=w510, error in=w512) -> (specific class reference=w504:refnum<vi>, error out=w506:errorcluster)
                                n160 = call "Struct Fill Cluster By Items Record.vi"("reinit cluster to default (false)"=FALSE, "error in"=w506, "data start offset (0)"=w502, "data in"=w503, "cluster ref (empty)"=w504) -> ("error out"=w505:errorcluster)  [unwired: 4 in, 2 out]
                              }
                            }
                          }
                          frame Default {
                            # "fail: invalid dimensions"
                          }
                        }
                        n161 = property class="Arr"(reference=w450, error in=w455, "Number of Columns"=w452, "Number of Rows"=w451) -> (error out=w454:errorcluster)  [unwired: 1 out]
                      }
                      frame 48, 50 {
                        w524 = refnum<vi> refnum  # Array
                        # "cast ref to general array"
                        # "lv: some kind of string"
                        n162 = To More Specific Class(target class=w524, reference=w526, error in=w525) -> (specific class reference=w519:refnum<vi>, error out=w520:errorcluster)
                        n163 = Multiply(x=w518, y=w517) -> (x*y=w516:i32)
                        n164 = case shown="1, 2" w521 {
                          selector: w521 -> [w533 _]
                          tunnel: [w531 w604] -> w514
                          tunnel: w523 -> [w541 _]
                          tunnel: w522 -> [w540 _]
                          tunnel: w517 -> [w539 _]
                          tunnel: w518 -> [w538 _]
                          tunnel: w520 -> [w536 w604]
                          tunnel: w519 -> [w530 _]
                          tunnel: w516 -> [w528 _]
                          tunnel: w515 -> [w527 _]
                          frame 1, 2 {
                            # "fail?"
                            # "1D/2D array - extract string array from octave data"
                            n165 = Reshape Array(w540, w538, w539) -> (w537:u32[][])
                            n166 = for {
                              shift-right: [w586] -> w532
                              shift-left: w536 -> [w585]
                              tunnel: w541 -> [w584]
                              tunnel: w537 -> [w583] mode=indexing
                              tunnel: [w582] -> w529 mode=indexing
                              tunnel: [w581] -> w535 mode=indexing
                              n167 = for {
                                shift-right: [w600] -> w586
                                shift-left: w585 -> [w603]
                                tunnel: w584 -> [w602]
                                tunnel: w583 -> [w601] mode=indexing
                                tunnel: [w596] -> w582 mode=indexing if=w587
                                tunnel: [w587] -> w581 mode=indexing
                                # "extract item of array"
                                # "item is part of cell array of strings"
                                n168 = call "Struct Parse Binary.vi"("error in"=w603, "data start offset (0)"=w601, "data in"=w602) -> ("error out"=w600:errorcluster, "struct items"=w599:T1[])  [unwired: 7 in]
                                n169 = Array Size(array=w599) -> (size(s)=w594:i32)
                                n170 = Index Array(array=w599) -> (element=w598:T1)  [unwired: 1 in]
                                n171 = Equal?(x=w594, y=1) -> (x = y?=w590:bool)
                                n172 = Unbundle By Name(w598) -> ("data"=w597:u8[], "name"=w591:string, "type"=w592:T2)
                                n173 = Byte Array To String(unsigned byte array=w597) -> (string=w596:string)
                                n174 = Empty String/Path?(string/path=w591) -> (empty?=w589:bool)
                                n175 = Equal?(x=w592, y=Struct_Item_Types."string") -> (x = y?=w588:bool)
                                n176 = Compound Arithmetic op=AND(w589, w588, w590) -> (w587:bool)
                              }
                            }
                            n177 = And Array Elements(Boolean array=w535) -> (logical AND=w534:bool)
                            n178 = case shown="True" w534 {
                              tunnel: w533 -> [_ w549]
                              tunnel: w532 -> [w542 w548]
                              tunnel: [w542 w547] -> w531
                              tunnel: w530 -> [_ w546]
                              tunnel: w529 -> [_ w545]
                              tunnel: w528 -> [_ w544]
                              tunnel: w527 -> [_ w543]
                              frame False {
                                # "fail - some items are not strings!"
                              }
                              frame True {
                                # "oukej - all items are strings"
                                n179 = case shown="2" w549 {
                                tunnel: w548 -> [w556 w571]
                                tunnel: [w555 w570] -> w547
                                tunnel: w546 -> [w554 w569]
                                tunnel: w545 -> [w553 w567]
                                tunnel: w544 -> [w552 _]
                                tunnel: w543 -> [w550 w568]
                                frame 1, Default {
                                # "1D"
                                n180 = Reshape Array(w553, w552) -> (w551:string[])
                                n181 = case shown="32" w550 {
                                tunnel: w556 -> [w560 w565]
                                tunnel: [w559 w564] -> w555
                                tunnel: w554 -> [w558 w563]
                                tunnel: w551 -> [w557 w562]
                                frame Default {
                                # "string"
                                n182 = property class="Arr"(reference=w558, error in=w560, "Value"=w557) -> (error out=w559:errorcluster)  [unwired: 1 out]
                                }
                                frame 50 {
                                # "path"
                                n183 = String To Path(string=w562) -> (path=w561:path[])
                                n184 = property class="Arr"(reference=w563, error in=w565, "Value"=w561) -> (error out=w564:errorcluster)  [unwired: 1 out]
                                }
                                }
                                }
                                frame 2 {
                                # "2D"
                                n185 = Transpose 2D Array(2D array=w567) -> (transposed array=w566:string[][])
                                n186 = case shown="32" w568 {
                                tunnel: w571 -> [w575 w580]
                                tunnel: [w574 w579] -> w570
                                tunnel: w569 -> [w573 w578]
                                tunnel: w566 -> [w572 w577]
                                frame Default {
                                # "string"
                                n187 = property class="Arr"(reference=w573, error in=w575, "Value"=w572) -> (error out=w574:errorcluster)  [unwired: 1 out]
                                }
                                frame 50 {
                                # "path"
                                n188 = String To Path(string=w577) -> (path=w576:path[][])
                                n189 = property class="Arr"(reference=w578, error in=w580, "Value"=w576) -> (error out=w579:errorcluster)  [unwired: 1 out]
                                }
                                }
                                }
                                }
                              }
                            }
                          }
                          frame Default {
                            # "fail: invalid dimensions"
                          }
                        }
                      }
                      frame Default {
                        # "invalid lv item type"
                      }
                    }
                  }
                }
              }
              frame "Cluster" {
                # "cluster"
                n190 = Equal?(x=w615, y=1) -> (x = y?=w610:bool)
                n191 = Equal?(x=w613, y=Struct_Item_Types."cell array") -> (x = y?=w611:bool)
                n192 = Compound Arithmetic op=AND(w610, w611) -> (w609:bool)
                n193 = case shown="True" w609 {
                  tunnel: w616 -> [w617 w623]
                  tunnel: w608 -> [_ w618]
                  tunnel: w607 -> [_ w621]
                  tunnel: [w617 w620] -> w606
                  frame False {
                    # "invalid octave data"
                  }
                  frame True {
                    w624 = refnum<vi> refnum  # Cluster
                    # "!!! recursion !!!"
                    # "convert ctrl ref\nto cluster ref"
                    # "octave: struct or cell array with one elemnt which is struct"
                    n194 = To More Specific Class(target class=w624, reference=w618, error in=w623) -> (specific class reference=w619:refnum<vi>, error out=w622:errorcluster)
                    n195 = call "Struct Fill Cluster By Items Record.vi"("error in"=w622, "data in"=w621, "cluster ref (empty)"=w619) -> ("error out"=w620:errorcluster)  [unwired: 6 in, 2 out]
                  }
                }
              }
              frame Default {
                # "unknown item"
              }
            }
          }
          frame -1 {
          }
        }
      }
    }
  }
  "error out" <- w9
  "cluster ref out (copy)" <- "cluster ref (empty)"
